vi "nanocal calculate.vi"(7 "nanocal calc command":T3, 9 "nanocal config":T4={"Hs"={"out"=enum."D", "shunt R (Ohm)"=100000.0, "V"={"c"=enum."A V1", "l"=enum."Lock-in set L1"}, "\"I\""={"c"=enum."A V2", "l"=enum."Lock-in set L1"}}, "ofset heater"={"out"=enum."C", "\"I\""=enum."C V2", "shunt R (Ohm)"=10000.0}, "Ts"={"out"=enum."D", "shunt R (Ohm)"=100000.0, "V"={"c"=enum."D V1", "l"=enum."Lock-in set L1"}, "\"I\""={"c"=enum."D V2", "l"=enum."Lock-in set L1"}}, "Tr"={"out"=enum."B", "shunt R (Ohm)"=100000.0, "V"={"c"=enum."E V1", "l"=enum."Lock-in set L1"}, "\"I\""={"c"=enum."E V2", "l"=enum."Lock-in set L1"}}, "Hr"={"out"=enum."E", "shunt R (Ohm)"=100000.0, "V"={"c"=enum."B V1", "l"=enum."Lock-in set L1"}, "\"I\""={"c"=enum."B V2", "l"=enum."Lock-in set L1"}}, "differential"={"c"=enum."C V1", "l"=enum."Lock-in set L2"}} {"Hr"."shunt R (Ohm)" format="%#_6p"; "Tr"."shunt R (Ohm)" format="%#_6p"; "Ts"."shunt R (Ohm)" format="%#_6p"; "ofset heater"."shunt R (Ohm)" format="%#_6p"; "Hs"."shunt R (Ohm)" format="%#_6p"}, 10 "engine reading":T2={"Ts -- V (V)"=100000.0+0.0i, "Hr -- V (V)"=100000.0+0.0i, "Hs -- V (V)"=100000.0+0.0i, "Tr -- V (V)"=100000.0+0.0i, "Diff -- V (V)"=100000.0+0.0i, "offset (V)"=100000.0+0.0i, "Ts -- \"I\" (V)"=100000.0+0.0i, "Hs -- \"I\" (V)"=100000.0+0.0i, "Tr -- \"I\" (V)"=100000.0+0.0i, "Hr -- \"I\" (V)"=100000.0+0.0i, "freq (Hz)"=100000.0} {"freq (Hz)" format="%#_6p"; "Hr -- \"I\" (V)" format="%#_6p"; "Tr -- \"I\" (V)" format="%#_6p"; "Hs -- \"I\" (V)" format="%#_6p"; "Ts -- \"I\" (V)" format="%#_6p"; "offset (V)" format="%#_6p"; "Diff -- V (V)" format="%#_6p"; "Tr -- V (V)" format="%#_6p"; "Hs -- V (V)" format="%#_6p"; "Hr -- V (V)" format="%#_6p"; "Ts -- V (V)" format="%#_6p"}, 11 "nanocal data array":T1[](array[typedef])) -> (1 "number":cdb)   [LabVIEW 2020]
uses:
  nanocal - config.ctl
  resistoricicle.ctl
  channelicicle.ctl
  NanoCalLib 20210521/MCL.lvlibp/SynkTek FPGA/FPGA_SharedResources/FPGASharedResources_Readings_ReadingChannelTypedef.ctl
  NanoCalLib 20210521/MCL.lvlibp/SynkTek FPGA/FPGA_SharedResources/FPGASharedResources_Lockin_Typedef.ctl
  nanocal calc command.ctl
  engine reading icicle.ctl
  icicle.ctl
  NanoCalLib 20210521/MCL.lvlibp/SynkTek FPGA/FPGA_SharedResources/FPGA_SharedResources.lvlib
panel:
  # "Ts"
  # "Tr"
  # "Hs"
  # "Hr"
  # "offset heater"
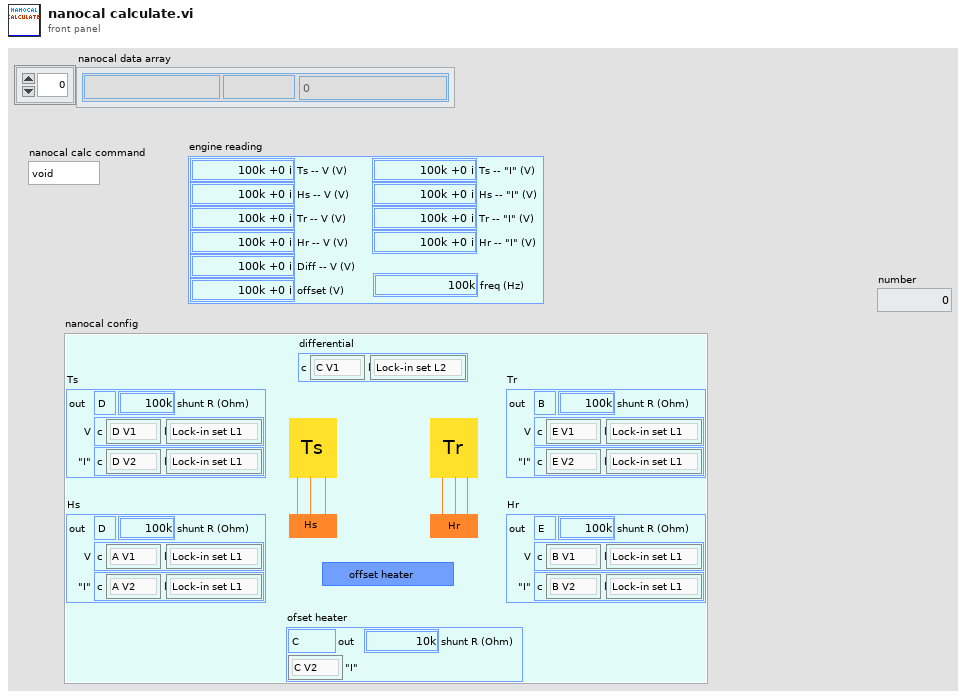
[diagram p1: front panel]
types:
  T1 = typedef "icicle.ctl" = cluster{"name":string, "units":string, "data":dbl}
  T2 = typedef "engine reading icicle.ctl" = cluster{"Ts -- V (V)":cdb, "Hr -- V (V)":cdb, "Hs -- V (V)":cdb, "Tr -- V (V)":cdb, "Diff -- V (V)":cdb, "offset (V)":cdb, "Ts -- \"I\" (V)":cdb, "Hs -- \"I\" (V)":cdb, "Tr -- \"I\" (V)":cdb, "Hr -- \"I\" (V)":cdb, "freq (Hz)":dbl}
  T3 = typedef "nanocal calc command.ctl" = enum16{"void", "R(omega)", "C/T (J/K^2)"}
  T4 = typedef "nanocal - config.ctl" = cluster{"Hs":T5, "ofset heater":cluster{"out":enum16{"A", "B", "C", "D", "E"}, "\"I\"":T7, "shunt R (Ohm)":dbl}, "Ts":T5, "Tr":T5, "Hr":T5, "differential":T6}
  T5 = typedef "resistoricicle.ctl" = cluster{"out":enum16{"A", "B", "C", "D", "E"}, "shunt R (Ohm)":dbl, "V":T6, "\"I\"":T6}
  T6 = typedef "channelicicle.ctl" = cluster{"c":T7, "l":T8}
  T7 = typedef "MCL.lvlibp/FPGA_SharedResources.lvlib/FPGASharedResources_Readings_ReadingChannelTypedef.ctl" = enum8{"A V1", "A V2", "B V1", "B V2", "C V1", "C V2", "D V1", "D V2", "E V1", "E V2", "A I", "B I", "C I", "D I", "E I", "Int."}
  T8 = typedef "MCL.lvlibp/FPGA_SharedResources.lvlib/FPGASharedResources_Lockin_Typedef.ctl" = enum8{"Lock-in set L1", "Lock-in set L2"}
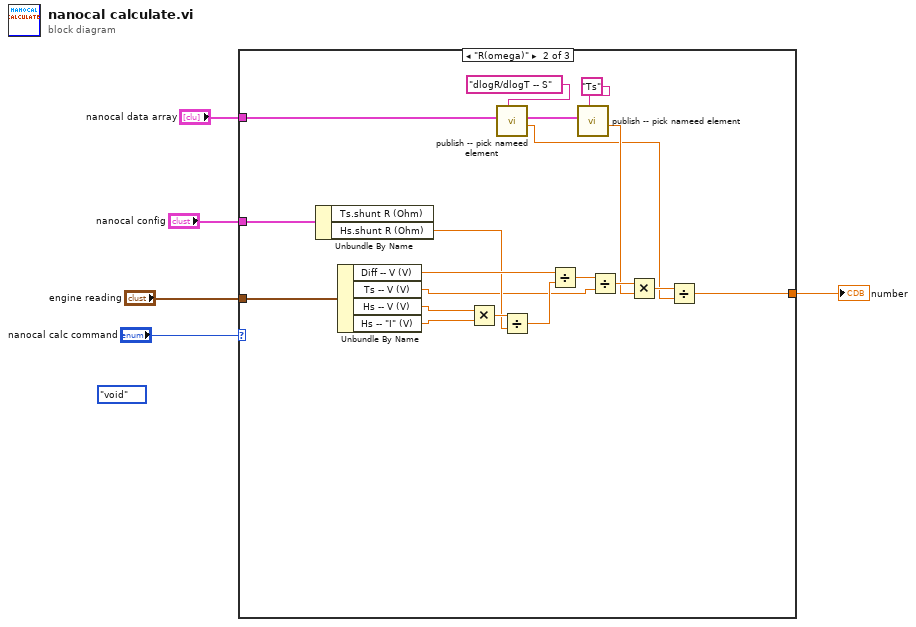
[diagram p0: block diagram]
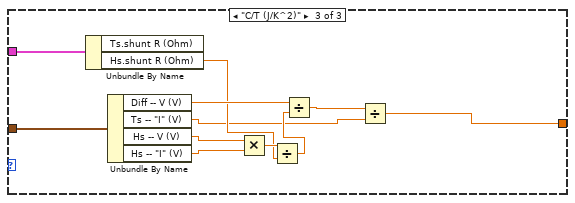
[diagram p3: hidden frame]
diagram:
  (unwired) nanocal_calc_command."void" ("nanocal calc command")
  n1 = case shown="\"R(omega)\"" "nanocal calc command" {
    tunnel: "nanocal config" -> [_ w24 w35]
    tunnel: "engine reading" -> [_ w23 w34]
    tunnel: [_ w8 w25] -> w2
    tunnel: "nanocal data array" -> [_ w13 _]
    frame "void", Default {
    }
    frame "R(omega)" {
      n2 = Unbundle By Name(w24) -> ("Hs.shunt R (Ohm)"=w18:dbl)  [unwired: 1 out]
      n3 = Unbundle By Name(w23) -> ("Diff -- V (V)"=w22:cdb, "Ts -- V (V)"=w15:cdb, "Hs -- V (V)"=w21:cdb, "Hs -- \"I\" (V)"=w20:cdb)
      n4 = Multiply(x=w21, y=w20) -> (x*y=w19:cdb)
      n5 = call "publish -- pick nameed element.vi"("name"="dlogR/dlogT -- S", "nanocal data array"=w13) -> ("element"=w9:dbl, "nanocal data array OUT"=w12:T1[])  [unwired: 8 in]
      n6 = Divide(x=w19, y=w18) -> (x/y=w17:cdb)
      n7 = Divide(x=w22, y=w17) -> (x/y=w16:cdb)
      n8 = call "publish -- pick nameed element.vi"("name"="Ts", "nanocal data array"=w12) -> ("element"=w11:dbl)  [unwired: 8 in, 1 out]
      n9 = Divide(x=w16, y=w15) -> (x/y=w14:cdb)
      n10 = Multiply(x=w14, y=w11) -> (x*y=w10:cdb)
      n11 = Divide(x=w10, y=w9) -> (x/y=w8:cdb)
    }
    frame "C/T (J/K^2)" {
      n12 = Unbundle By Name(w35) -> ("Hs.shunt R (Ohm)"=w29:dbl)  [unwired: 1 out]
      n13 = Unbundle By Name(w34) -> ("Diff -- V (V)"=w33:cdb, "Ts -- \"I\" (V)"=w26:cdb, "Hs -- V (V)"=w32:cdb, "Hs -- \"I\" (V)"=w31:cdb)
      n14 = Multiply(x=w32, y=w31) -> (x*y=w30:cdb)
      n15 = Divide(x=w30, y=w29) -> (x/y=w28:cdb)
      n16 = Divide(x=w33, y=w28) -> (x/y=w27:cdb)
      n17 = Divide(x=w27, y=w26) -> (x/y=w25:cdb)
    }
  }
  "number" <- w2
